vi "solar_voy_def Quotes Add Desc.vi"(11 "Description":string) -> (3 "Description with Comments":string)   [LabVIEW 2018]
doc: "This adds quotes to a description."
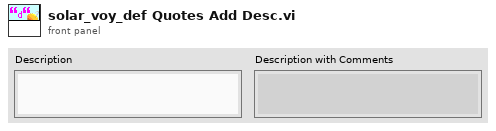
[diagram p1: front panel]
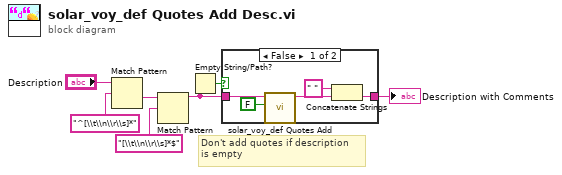
[diagram p0: block diagram]
diagram:
  # "Don't add quotes if description\nis empty"
  n1 = Match Pattern(string="Description", regular expression="^[\\t\\n\\r\\s]*") -> (after substring=w3:string)  [unwired: 1 in, 3 out]
  n2 = Match Pattern(string=w3, regular expression="[\\t\\n\\r\\s]*$") -> (before substring=w5:string)  [unwired: 1 in, 3 out]
  n3 = Empty String/Path?(string/path=w5) -> (empty?=w4:bool)
  n4 = case shown="False" w4 {
    tunnel: [w9 w13] -> w6
    tunnel: w5 -> [w10 w13]
    frame False {
      n5 = call "solar_voy_def Quotes Add.vi"("Whitespace Only? (F=Always)"=FALSE ("Add Comments if Empty? (T)"), "String"=w10) -> ("String with Comments"=w11:string)  [unwired: 9 in]
      n6 = Concatenate Strings(" " ("string"), w11) -> (w9:string)
    }
    frame True {
    }
  }
  "Description with Comments" <- w6
